vi "Mischverhaeltnis.vi"(8 "error in (no error)":errorcluster caption="Fehler (Eingang, kein Fehler)", 9 "Konzentration":dbl, 11 "Sollwert":dbl) -> (0 "error out":errorcluster caption="Fehler (Ausgang)", 3 "%":dbl)   [LabVIEW 2020, in "Linearisierung v2.lvlib" / "Gasteiler.lvlib" / "HovaCal.lvlib"]
uses:
  HovaCal.lvlib
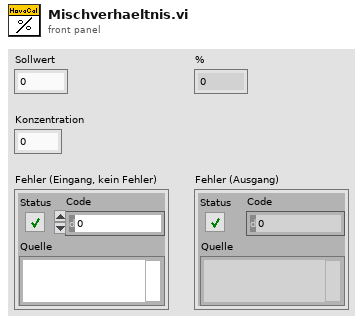
[diagram p1: front panel]
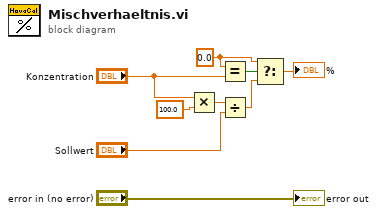
[diagram p0: block diagram]
diagram:
  w4 = 0.0 ("x")
  n1 = Multiply(x="Konzentration", y=100.0) -> (x*y=w8:dbl)
  n2 = Equal?(x=w4, y="Konzentration") -> (x = y?=w5:bool)
  n3 = Divide(x=w8, y="Sollwert") -> (x/y=w6:dbl)
  n4 = Select(t=w4, s=w5, f=w6) -> (s? t:f=→"%":dbl)
  "error out" <- "error in (no error)"
